vi "Read Interrupts HW.vi"(8 "error in (no error)":errorcluster, 11 "BME_DG_System in":refnum<class "BME_DG_System.lvclass">) -> (0 "error out":errorcluster, 2 "Interrupts":u32[](array[numeric]), 3 "BME_DG_System out":refnum<class "BME_DG_System.lvclass">)   [LabVIEW 2009, in "POLARIS BME DG.lvlib" / "BME_DG_System.lvclass"]
uses:
  BME_DG_System.lvclass
  BME_DG_System.lvclass/BME_DG_System.ctl
  BME_DG_Base/BME_DG_Base.lvclass
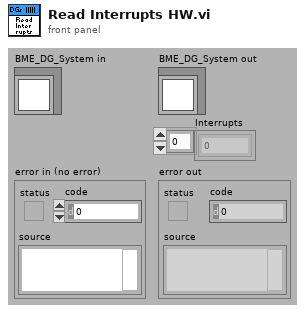
[diagram p1: front panel]
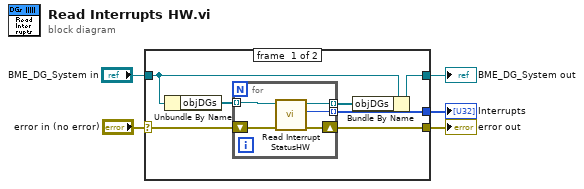
[diagram p0: block diagram]
diagram:
  n1 = case shown="No Error" "error in (no error)" {
    selector: "error in (no error)" -> [w10 w19]
    tunnel: [w9 w19] -> w4
    tunnel: [w8 w18] -> w2
    tunnel: "BME_DG_System in" -> [w12 w18]
    tunnel: [w6 _] -> w1
    frame #0 {
      n2 = Unbundle By Name(w12) -> ("objDGs"=w11:refnum<class "BME_DG_Base.lvclass">[])
      n3 = for {
        tunnel: w11 -> [w17] mode=indexing
        tunnel: [w15] -> w7 mode=indexing
        shift-right: [w13] -> w9
        shift-left: w10 -> [w16]
        tunnel: [w14] -> w6 mode=indexing
        n4 = call-dynamic "Read Interrupt StatusHW.vi"("error in (no error)"=w16, "BME_DG_Base in"=w17) -> ("error out"=w13:errorcluster, "Interrupt Status"=w14:u32, "BME_DG_Base out"=w15:refnum<class "BME_DG_Base.lvclass">)  [unwired: 7 in]
      }
      n5 = Bundle By Name(cluster=w12, "objDGs"=w7) -> (w8:refnum<class "BME_DG_System.lvclass">)
    }
    frame #1 {
    }
  }
  "error out" <- w4
  "BME_DG_System out" <- w2
  "Interrupts" <- w1
